vi "set_smith_cursor_plot.vi"(6 "path":path, 7 "smith_plot":refnum<vi>, 8 "cursor_pos":i32, 9 "cursor_index":i32, 11 "plot_rjx":cluster{"array type (2D Dbl)":dbl[], dbl[]}[](array[cluster])) -> ()   [LabVIEW 2025]
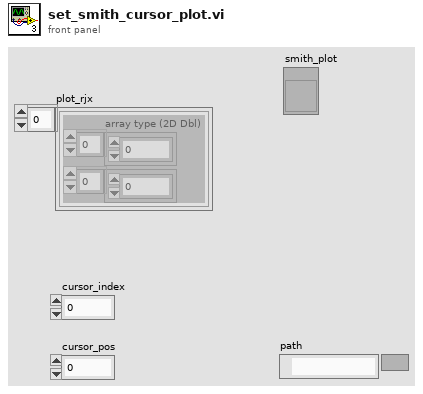
[diagram p1: front panel]
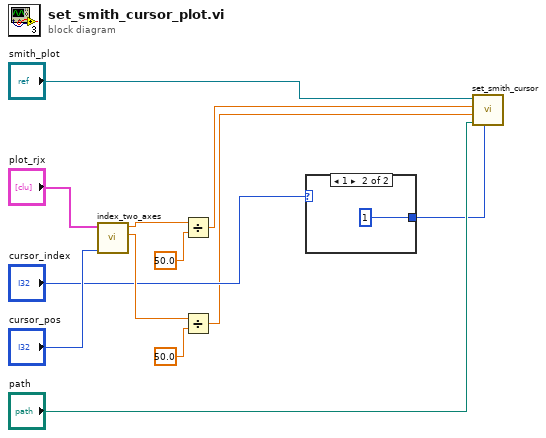
[diagram p0: block diagram]
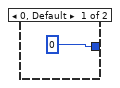
[diagram p2: hidden frame]
diagram:
  n1 = call "index_two_axes.vi"("x_index"="cursor_pos", "graph_data"="plot_rjx") -> ("Y2"=w12:dbl, "Y1"=w11:dbl)  [unwired: 7 in, 1 out]
  n2 = Divide(x=w11, y=50.0) -> (x/y=w5:dbl)
  n3 = Divide(x=w12, y=50.0) -> (x/y=w1:dbl)
  n4 = case shown="1" "cursor_index" {
    tunnel: [0 ("deco_id") 1 ("deco_id")] -> w2
    frame 0, Default {
    }
    frame 1 {
    }
  }
  n5 = call "set_smith_cursor.vi"("deco_id"=w2, "vi path"="path", "x"=w1, "r"=w5, "show_plot_ref"="smith_plot") -> ()  [unwired: 7 in]
